vi "test-trapezoid-profile-switch-goal-in-middle.vi"() -> (3 "Test Passed":bool)   [LabVIEW 2019]
uses:
  <vilib>/Rock Robotics/WPI/ThirdParty/JAS_Junk/TrajLib/TRAPEZOID_PROFILE_STATE.ctl
  <vilib>/Rock Robotics/WPI/ThirdParty/JAS_Junk/TrajLib/TRAPEZOID_PROFILE.ctl
  <vilib>/Rock Robotics/WPI/ThirdParty/JAS_Junk/TrajLib/TRAPEZOID_PROFILE_CONSTRAINT.ctl
  <vilib>/Rock Robotics/WPI/ThirdParty/JAS_Junk/TrajLib/TrapProfile_ShouldFlipAcceleration.vi
  <vilib>/Rock Robotics/WPI/ThirdParty/JAS_Junk/TrajLib/TrapProfile_Direct.vi
  <vilib>/Rock Robotics/SystemInterfaces/NetworkCommunication/NetComm_UsageReport_report.vi
  <vilib>/Rock Robotics/WPI/ThirdParty/JAS_Junk/TrajLib/Util_LibraryGlobals.vi
  <vilib>/Rock Robotics/WPI/ThirdParty/JAS_Junk/TrajLib/Trajectory_Library.lvlib
panel:
  out "Goal":T1 {"Velocity" format="%16_6e"; "Position" format="%16_6e"}
  out "ApproxEquals 2":bool
  out "ApproxEquals":bool
  out "Equal":bool
  out "State 2":T1 {"Velocity" format="%16_6e"; "Position" format="%16_6e"}
  out "Waveform Chart 2":T2(graph)
  out "TRAPEZOID_PROFILE 2":T3 {"Goal"."Velocity" format="%16_6e"; "Goal"."Position" format="%16_6e"; "Initial"."Velocity" format="%16_6e"; "Initial"."Position" format="%16_6e"; "Constraints"."MaxAcceleration" format="%16_6e"; "Constraints"."MaxVelocity" format="%16_6e"; "EndDecel" format="%16_6e"; "EndFullSpeed" format="%16_6e"; "EndAccel" format="%16_6e"}
  out "TRAPEZOID_PROFILE":T3 {"Goal"."Velocity" format="%16_6e"; "Goal"."Position" format="%16_6e"; "Initial"."Velocity" format="%16_6e"; "Initial"."Position" format="%16_6e"; "Constraints"."MaxAcceleration" format="%16_6e"; "Constraints"."MaxVelocity" format="%16_6e"; "EndDecel" format="%16_6e"; "EndFullSpeed" format="%16_6e"; "EndAccel" format="%16_6e"}
  out "State":T1 {"Velocity" format="%16_6e"; "Position" format="%16_6e"}
  out "Waveform Chart":T2(graph)
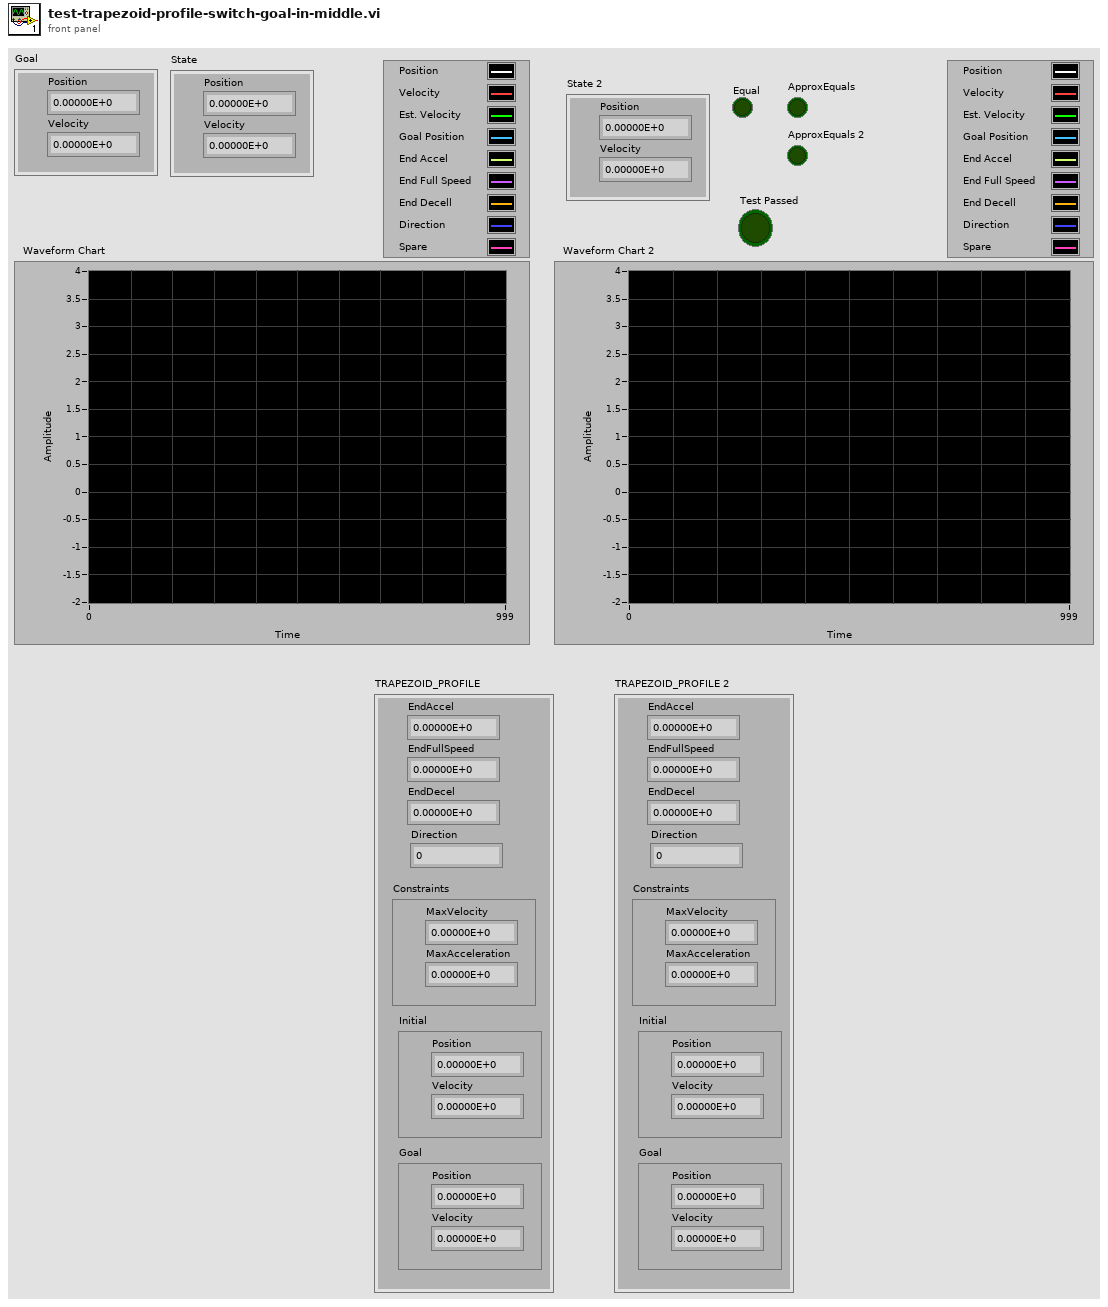
[diagram p1: front panel]
types:
  T1 = typedef "Trajectory_Library.lvlib/TRAPEZOID_PROFILE_STATE.ctl" = cluster{"Position":dbl, "Velocity":dbl}
  T2 = cluster{"Position":dbl, "Velocity":dbl, dbl, "Position":dbl, "EndAccel":dbl, "EndFullSpeed":dbl, "EndDecel":dbl, "Direction":i32, "Position":dbl}
  T3 = typedef "Trajectory_Library.lvlib/TRAPEZOID_PROFILE.ctl" = cluster{"EndAccel":dbl, "EndFullSpeed":dbl, "EndDecel":dbl, "Direction":i32, "Constraints":T4, "Initial":T1, "Goal":T1}
  T4 = typedef "Trajectory_Library.lvlib/TRAPEZOID_PROFILE_CONSTRAINT.ctl" = cluster{"MaxVelocity":dbl, "MaxAcceleration":dbl}
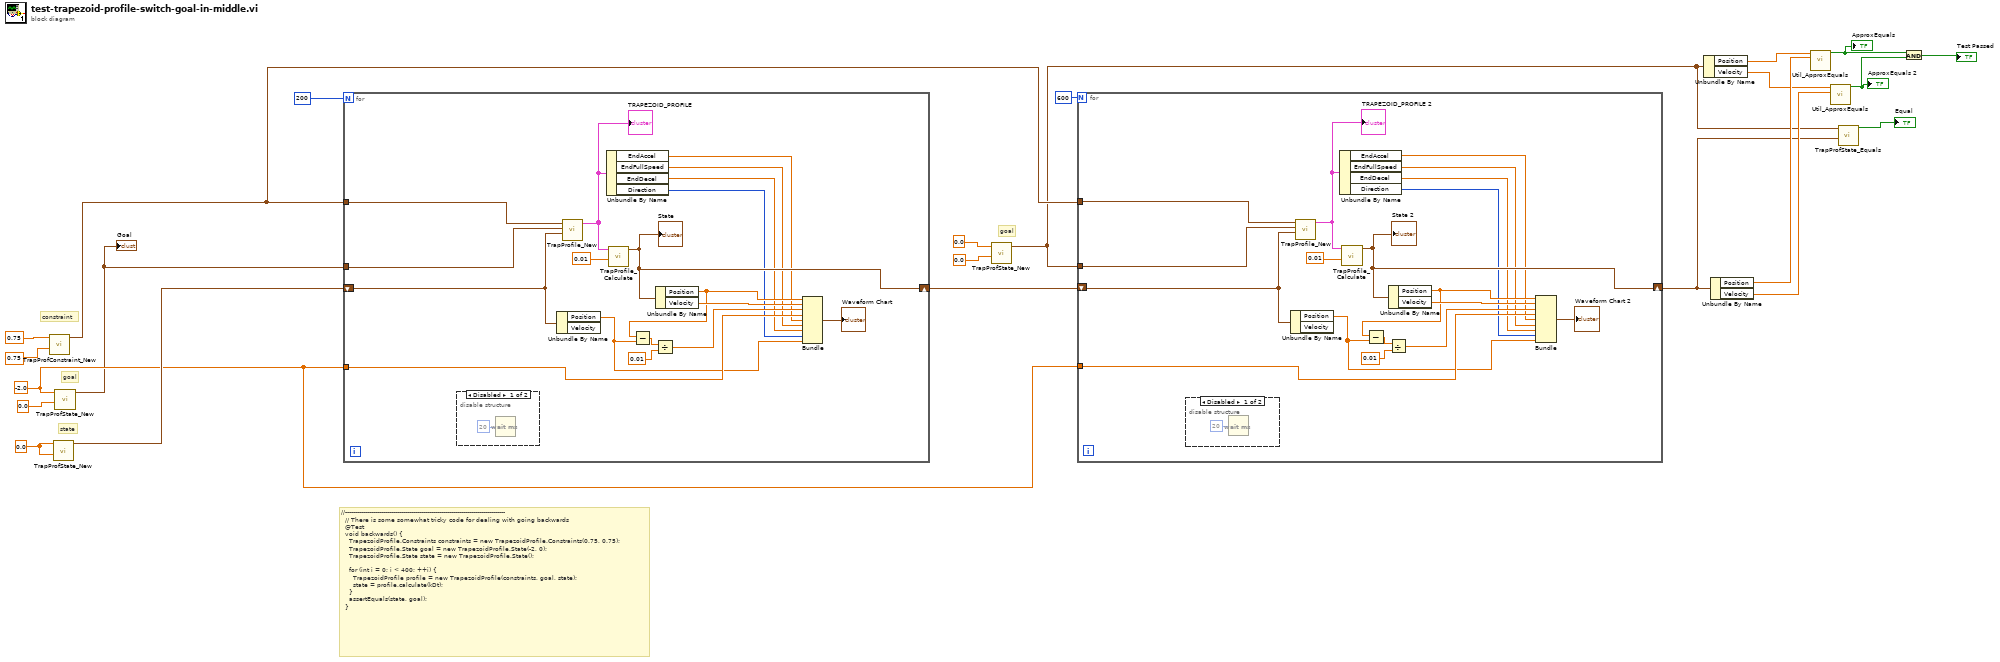
[diagram p0: block diagram]
diagram:
  w19 = 0.0 ("Position")
  w12 = -2.0 ("Position")
  # "goal"
  # "state"
  # "//--------------------------------------------------------------------------------\n  // There is some somewhat tricky code for dealing with going backwards\n  @Test\n  void backwards() {\n    TrapezoidProfile.Constraints constraints = new TrapezoidProfile.Constraints(0.75, 0.75);\n    TrapezoidProfile.State goal = new TrapezoidProfile.State(-2, 0);\n    TrapezoidProfile.State state = new TrapezoidProfile.State();\n\n    for (int i = 0; i < 400; ++i) {\n      TrapezoidProfile profile = new TrapezoidProfile(constraints, goal, state);\n      state = profile.calculate(kDt);\n    }\n    assertEquals(state, goal);\n  }"
  # "goal"
  # "constraint"
  n1 = call <vilib>:"TrapProfConstraint_New.vi"("Max Accel"=0.75, "Max Speed (M/S)"=0.75) -> ("TRAPEZOID_PROFILE_CONSTRAINT"=w13:T4)  [unwired: 9 in]
  n2 = call <vilib>:"TrapProfState_New.vi"("Velocity"=w19, "Position"=w19) -> ("TRAPEZOID_PROFILE_STATE"=w18:T1)  [unwired: 9 in]
  n3 = call <vilib>:"TrapProfState_New.vi"("Velocity"=0.0, "Position"=w12) -> ("TRAPEZOID_PROFILE_STATE"=w2:T1)  [unwired: 9 in]
  "Goal" <- w2
  n4 = for {
    N: 200 -> [_]
    shift-right: [w32] -> w14
    shift-left: w18 -> [w37]
    tunnel: w2 -> [w39]
    tunnel: w12 -> [w31]
    tunnel: w13 -> [w24]
    n5 = disable-structure shown="Disabled" {
      frame Disabled {
        n6 = Wait (ms)(milliseconds to wait=u32 20) -> ()  [unwired: 1 out]
      }
      frame Enabled {
      }
    }
    n7 = Unbundle By Name(w37) -> ("Position"=w25:dbl)  [unwired: 1 out]
    n8 = call <vilib>:"TrapProfile_New.vi"("Initial"=w37, "Goal"=w39, "Constraints"=w24) -> ("TRAPEZOID_PROFILE"=w30:T3)  [unwired: 8 in]
    "TRAPEZOID_PROFILE" <- w30
    n9 = Unbundle By Name(w30) -> ("EndAccel"=w29:dbl, "EndFullSpeed"=w28:dbl, "EndDecel"=w27:dbl, "Direction"=w26:i32)
    n10 = call <vilib>:"TrapProfile_Calculate.vi"("Time"=0.01, "TRAPEZOID_PROFILE"=w30) -> ("State"=w32:T1)  [unwired: 9 in]
    "State" <- w32
    n11 = Unbundle By Name(w32) -> ("Position"=w36:dbl, "Velocity"=w40:dbl)
    n12 = Subtract(x=w36, y=w25) -> (x-y=w35:dbl)
    n13 = Divide(x=w35, y=0.01) -> (x/y=w33:dbl)
    n14 = Bundle("Position"=w36, "Velocity"=w40, w33, "Position"=w31, "EndAccel"=w29, "EndFullSpeed"=w28, "EndDecel"=w27, "Direction"=w26, "Position"=w25) -> (→"Waveform Chart":T2)  [unwired: 1 in]
  }
  n15 = call <vilib>:"TrapProfState_New.vi"("Velocity"=0.0, "Position"=0.0) -> ("TRAPEZOID_PROFILE_STATE"=w1:T1)  [unwired: 9 in]
  n16 = for {
    N: 600 -> [_]
    shift-right: [w51] -> w3
    shift-left: w14 -> [w56]
    tunnel: w1 -> [w58]
    tunnel: w12 -> [w50]
    tunnel: w13 -> [w43]
    n17 = disable-structure shown="Disabled" {
      frame Disabled {
        n18 = Wait (ms)(milliseconds to wait=u32 20) -> ()  [unwired: 1 out]
      }
      frame Enabled {
      }
    }
    n19 = Unbundle By Name(w56) -> ("Position"=w44:dbl)  [unwired: 1 out]
    n20 = call <vilib>:"TrapProfile_New.vi"("Initial"=w56, "Goal"=w58, "Constraints"=w43) -> ("TRAPEZOID_PROFILE"=w49:T3)  [unwired: 8 in]
    "TRAPEZOID_PROFILE 2" <- w49
    n21 = Unbundle By Name(w49) -> ("EndAccel"=w48:dbl, "EndFullSpeed"=w47:dbl, "EndDecel"=w46:dbl, "Direction"=w45:i32)
    n22 = call <vilib>:"TrapProfile_Calculate.vi"("Time"=0.01, "TRAPEZOID_PROFILE"=w49) -> ("State"=w51:T1)  [unwired: 9 in]
    "State 2" <- w51
    n23 = Unbundle By Name(w51) -> ("Position"=w55:dbl, "Velocity"=w59:dbl)
    n24 = Subtract(x=w55, y=w44) -> (x-y=w54:dbl)
    n25 = Divide(x=w54, y=0.01) -> (x/y=w52:dbl)
    n26 = Bundle("Position"=w55, "Velocity"=w59, w52, "Position"=w50, "EndAccel"=w48, "EndFullSpeed"=w47, "EndDecel"=w46, "Direction"=w45, "Position"=w44) -> (→"Waveform Chart 2":T2)  [unwired: 1 in]
  }
  n27 = Unbundle By Name(w1) -> ("Position"=w11:dbl, "Velocity"=w9:dbl)
  n28 = Unbundle By Name(w3) -> ("Position"=w10:dbl, "Velocity"=w7:dbl)
  n29 = call <vilib>:"Util_ApproxEquals.vi"("Value 2"=w10, "Value 1"=w11) -> ("ApproxEquals"=w5:bool)  [unwired: 9 in]
  "ApproxEquals" <- w5
  n30 = call <vilib>:"Util_ApproxEquals.vi"("Value 2"=w7, "Value 1"=w9) -> ("ApproxEquals"=w4:bool)  [unwired: 9 in]
  "ApproxEquals 2" <- w4
  n31 = call <vilib>:"TrapProfState_Equals.vi"("TRAPEZOID_PROFILE_STATE 2"=w3, "TRAPEZOID_PROFILE_STATE"=w1) -> ("Equal"=→"Equal":bool)  [unwired: 9 in]
  n32 = And(x=w5, y=w4) -> (x .and. y?=→"Test Passed":bool)
